vi "Demo.vi"() -> ()   [LabVIEW 2018]
uses:
  lib/Snap7.lvlib
panel:
  out "data out":string
  out "data string":string
  in  "?":bool
  out "time":u32
  in  "DB Number":i32=1
  in  "Start":i32
  in  "Amount":i32=16
  in  "Area":i32(ring)=132 items=["Inputs (EB)"=129, "Output (AB)"=130, "Bit Memory (M)"=131, "Data (DB)"=132, "Counters (Z)"=28, "Timers (T)"=29]
  in  "Word Length":i32(ring)=2 items=["Bit"=1, "Byte"=2, "Word"=4, "DWord"=6, "Real"=8, "Counter"=28, "Timer"=29]
  out "Running":bool
  out "Status":string="No Error"
  in  "Address IP":string="192.168.1.12"
  in  "Rack":i32
  in  "Slot":i32=2
  out "?":string
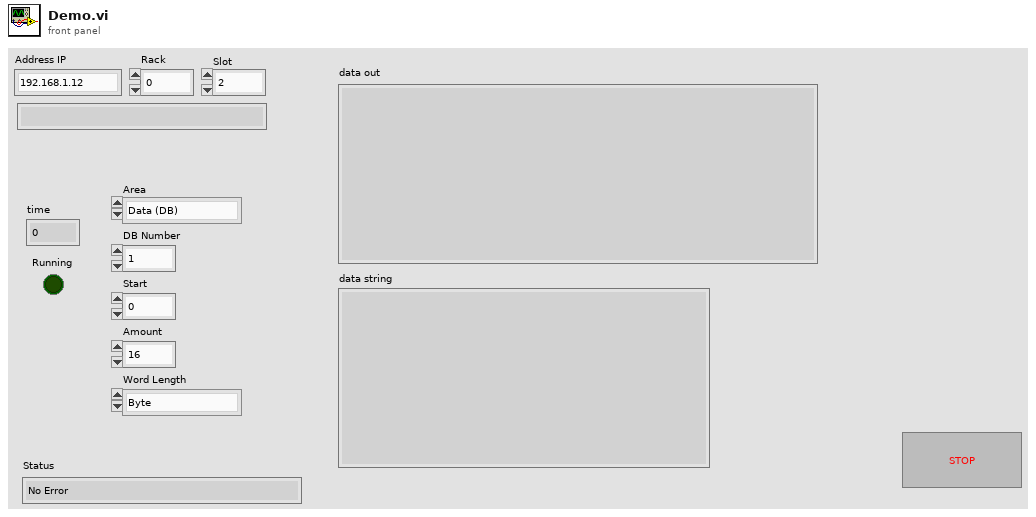
[diagram p1: front panel]
types:
  T1 = enum16{"big-endian, network order", "native, host order", "little-endian"}
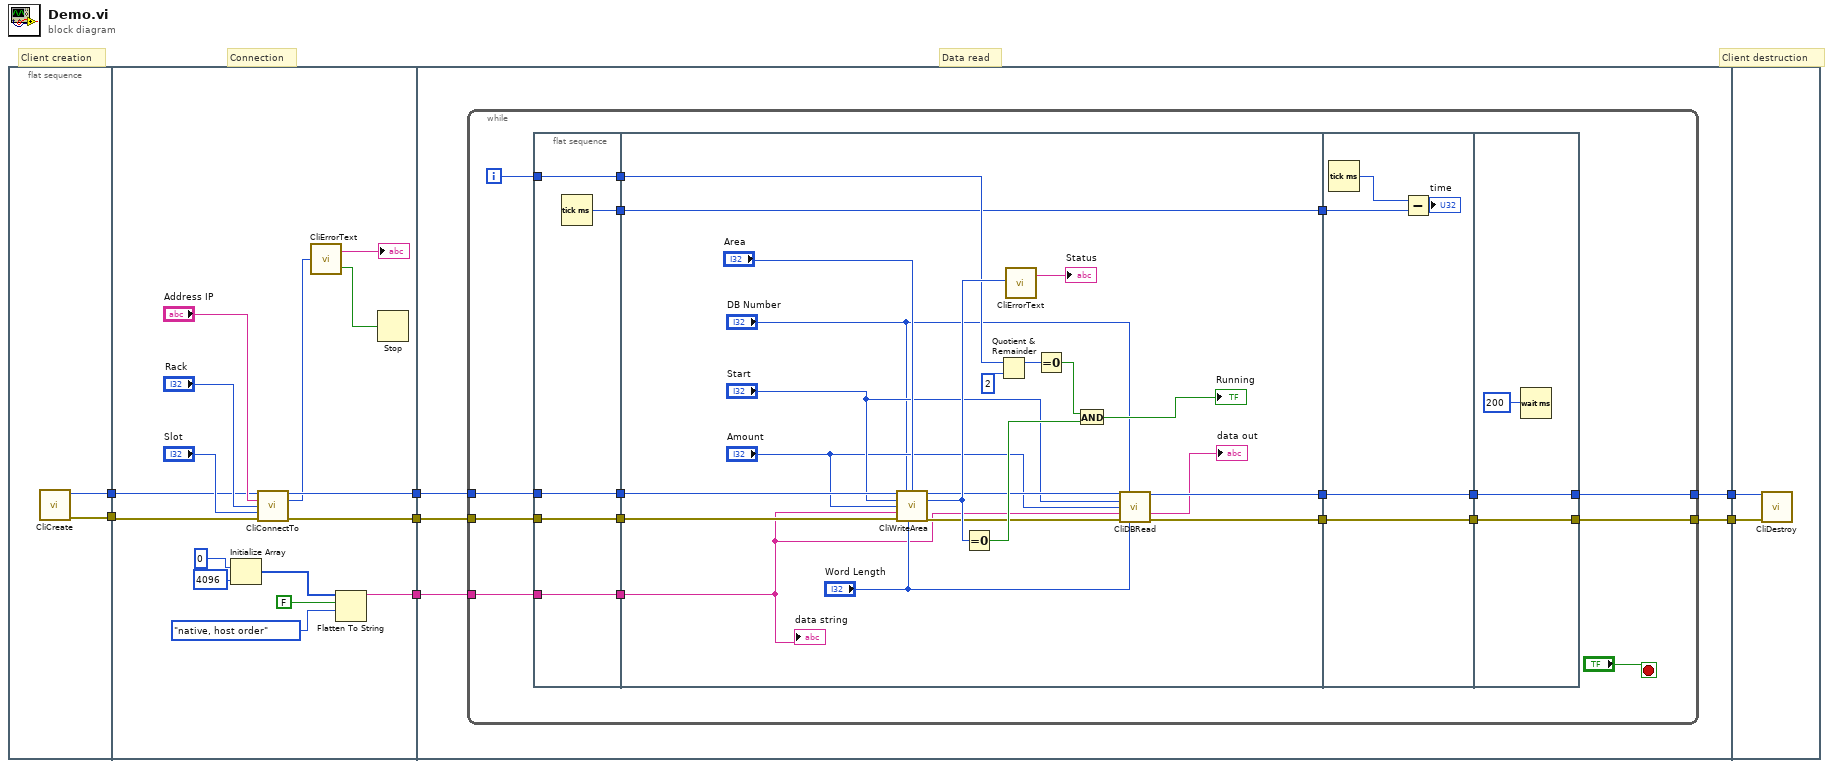
[diagram p0: block diagram]
diagram:
  # "Client destruction"
  # "Data read"
  # "Connection"
  # "Client creation"
  n1 = flat-sequence {
    tunnel: [w9] -> w7
    tunnel: [w8] -> w6
    tunnel: [w20] -> w5
    tunnel: [w13] -> w4
    tunnel: [w19] -> w3
    tunnel: w7 -> [w15]
    tunnel: w6 -> [w14]
    tunnel: w5 -> [w30]
    tunnel: w4 -> [w29]
    tunnel: w3 -> [w28]
    tunnel: [w27] -> w2
    tunnel: [w26] -> w1
    tunnel: w2 -> [w84]
    tunnel: w1 -> [w83]
    frame #0 {
      n2 = call "CliCreate.vi"() -> ("ref out"=w9:u64, "error out"=w8:errorcluster)  [unwired: 14 in]
    }
    frame #1 {
      n3 = Initialize Array(u8 0, 4096) -> (w23:u8[])
      n4 = call "CliConnectTo.vi"("ref in"=w15, "Address"="Address IP", "Rack"="Rack", "Slot"="Slot", "error in (no error)"=w14) -> ("ref out"=w13:u64, "Result"=w10:i32, "error out"=w20:errorcluster)  [unwired: 8 in]
      n5 = call "CliErrorText.vi"("ErrNo"=w10) -> ("Error"=w11:bool, "ErrMessage"=→"?":string)
      n6 = Flatten To String(anything=w23, prepend array or string size? (T)=FALSE, byte order (0:big-endian, network order)=T1."native, host order") -> (data string=w19:string)  [unwired: 1 in, 2 out]
      n7 = Stop(stop? (T)=w11) -> ()
    }
    frame #2 {
      n8 = while {
        tunnel: w30 -> [w46]
        tunnel: w29 -> [w45]
        tunnel: w28 -> [w44]
        tunnel: [w43] -> w27
        tunnel: [w42] -> w26
        i -> [w41]
        stop <- "?" stop-if-true
        n9 = flat-sequence {
          tunnel: w41 -> [w49]
          tunnel: w44 -> [w50]
          tunnel: w45 -> [w51]
          tunnel: w46 -> [w52]
          tunnel: [w52] -> w40
          tunnel: [w51] -> w39
          tunnel: [w50] -> w38
          tunnel: [w49] -> w37
          tunnel: [w48] -> w33
          tunnel: [w60] -> w35
          tunnel: w40 -> [w74]
          tunnel: w39 -> [w73]
          tunnel: w38 -> [w53]
          tunnel: w37 -> [w70]
          tunnel: w33 -> [w63]
          tunnel: [w63] -> w32
          tunnel: [w59] -> w31
          tunnel: [w79] -> w36
          tunnel: w35 -> [w78]
          tunnel: [w78] -> w34
          tunnel: w32 -> [w75]
          tunnel: w31 -> [w79]
          tunnel: [w81] -> w42
          tunnel: [w82] -> w43
          tunnel: w36 -> [w82]
          tunnel: w34 -> [w81]
          frame #0 {
            n10 = Tick Count (ms)() -> (millisecond timer value=w48:u32)
          }
          frame #1 {
            n11 = call "CliWriteArea.vi"("ref in"=w73, "DB Number"="DB Number", "Area"="Area", "Start"="Start", "Amount"="Amount", "data in"=w53, "error in (no error)"=w74, "Word Length"="Word Length") -> ("ref out"=w62:u64, "Result"=w71:i32, "error out"=w61:errorcluster)  [unwired: 5 in]
            n12 = Equal To 0?(x=w71) -> (x = 0?=w65:bool)
            n13 = Quotient & Remainder(x=w70, y=2) -> (x-y*floor(x/y)=w68:i32)  [unwired: 1 out]
            n14 = call "CliErrorText.vi"("ErrNo"=w71) -> ("ErrMessage"=→"Status":string)  [unwired: 1 out]
            n15 = Equal To 0?(x=w68) -> (x = 0?=w67:bool)
            n16 = And(x=w67, y=w65) -> (x .and. y?=→"Running":bool)
            n17 = call "CliDBRead.vi"("ref in"=w62, "DB Number"="DB Number", "Start"="Start", "Amount"="Amount", "data in"=w53, "error in (no error)"=w61, "Word Length"="Word Length") -> ("ref out"=w59:u64, "data out"=→"data out":string, "error out"=w60:errorcluster)  [unwired: 5 in, 1 out]
            "data string" <- w53
          }
          frame #2 {
            n18 = Tick Count (ms)() -> (millisecond timer value=w76:u32)
            n19 = Subtract(x=w76, y=w75) -> (x-y=→"time":u32)
          }
          frame #3 {
            n20 = Wait (ms)(milliseconds to wait=u32 200 ("Loop Delay (ms)")) -> ()  [unwired: 1 out]
          }
        }
      }
    }
    frame #3 {
      n21 = call "CliDestroy.vi"("ref in"=w84, "error in (no error)"=w83) -> ()  [unwired: 13 in, 1 out]
    }
  }
